vi "test2.vi"() -> ()   [LabVIEW 2023]
uses:
  <vilib>/userDefined/High Color/IMAQdx.ctl
  <vilib>/vision/driver/NI_Vision_Acquisition_Software.lvlib
  <resource>/objmgr/imaqdx.rc
panel:
  out "Bits Per Pix":u32
  out "Type of Img":u32
  out "Height":u32
  out "Width":u32
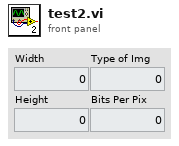
[diagram p1: front panel]
types:
  T1 = typedef "IMAQdx.ctl" = refnum<k21>
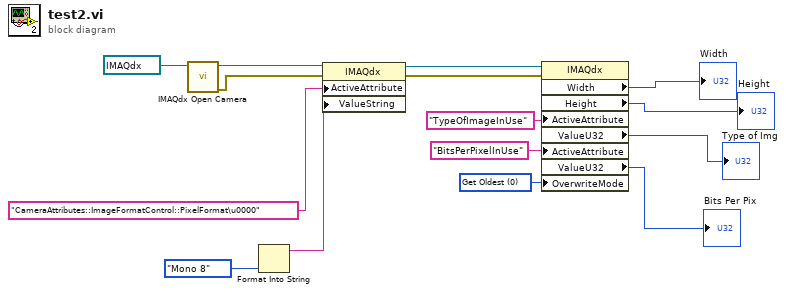
[diagram p0: block diagram]
diagram:
  w13 = u32 0 items=["Get Oldest"=0, "Fail"=2, "Get Newest"=3] ("OverwriteMode")
  n1 = call <vilib>:"IMAQdx Open Camera.vi"("Session In"=T1 "cam0") -> ("error out"=w5:errorcluster, "Session Out"=w6:T1)  [unwired: 2 in, 7 out]
  n2 = Format Into String(enum16{"Mono 10 p", "Mono 8", "Mono 10"}."Mono 8") -> (resulting string=w9:string)  [unwired: 3 in, 1 out]
  n3 = property class="IMAQdx"(reference=w6, error in=w5, "ActiveAttribute"="CameraAttributes::ImageFormatControl::PixelFormat\u0000", "ValueString"=w9) -> (reference out=w8:T1, error out=w7:errorcluster)
  n4 = property class="IMAQdx"(reference=w8, error in=w7, "ActiveAttribute"="TypeOfImageInUse", "ActiveAttribute"="BitsPerPixelInUse", "OverwriteMode"=w13) -> ("Width"=→"Width":u32, "Height"=→"Height":u32, "ValueU32"=→"Type of Img":u32, "ValueU32"=→"Bits Per Pix":u32)  [unwired: 2 out]
